vi "Set Session.vi"(8 "error in (no error)":errorcluster, 10 "ftp session":T1, 11 "FTP in":refnum<class "FTP.lvclass">) -> (0 "error out":errorcluster, 3 "FTP out":refnum<class "FTP.lvclass">)   [LabVIEW 2016, in "RT Management.lvlib" / "FTP.lvclass"]
uses:
  FTP.lvclass
  <vilib>/FTP/ftp0.llb/FTP Session.ctl
  FTP.lvclass/FTP.ctl
  <vilib>/FTP/NI_FTP.lvlib
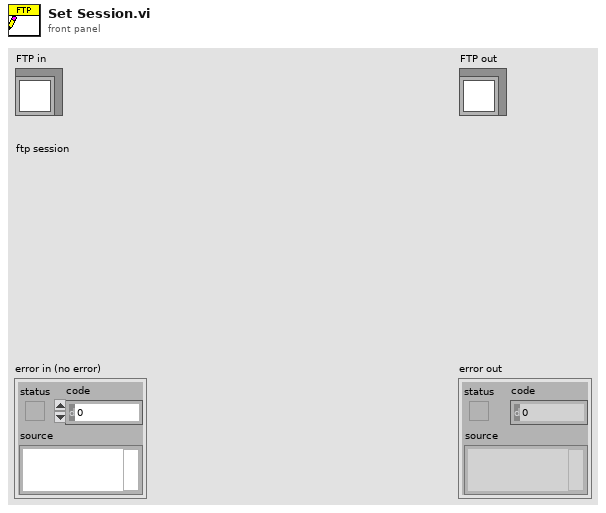
[diagram p1: front panel]
types:
  T1 = typedef "NI_FTP.lvlib/FTP Session.ctl" = refnum<k5>
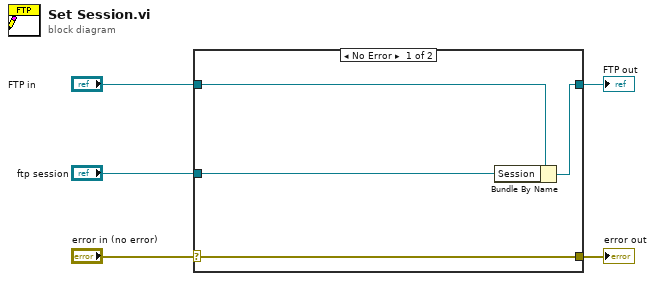
[diagram p0: block diagram]
diagram:
  n1 = case shown="No Error" "error in (no error)" {
    selector: "error in (no error)" -> [w9 w10]
    tunnel: [w9 w10] -> w4
    tunnel: [w7 w11] -> w2
    tunnel: "FTP in" -> [w8 w11]
    tunnel: "ftp session" -> [w6 _]
    frame No Error {
      n2 = Bundle By Name(cluster=w8, "Session"=w6) -> (w7:refnum<class "FTP.lvclass">)
    }
    frame Error {
    }
  }
  "error out" <- w4
  "FTP out" <- w2
